vi "Word_OpenReference.vi"(5 "Template File Path":string="C:\\Teststand\\LVFiles\\Support\\Sertifika_Format.dotx", 7 "File Visible ?":bool=TRUE, 8 "error in (no error)":errorcluster) -> (0 "error out":errorcluster, 3 "report out":refnum<class "NI_report.lvclass">)   [LabVIEW 2014]
doc: "This VI demonstrates the use of ActiveX to write a table into a Microsoft Excel worksheet."
uses:
  <vilib>/Utility/NIReport.llb/NI_report.lvclass
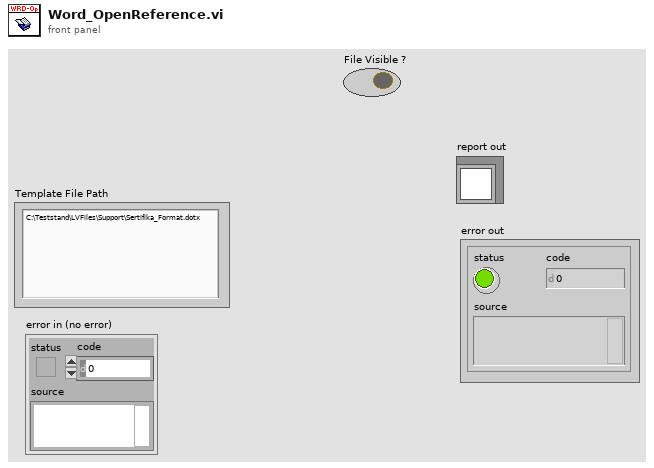
[diagram p1: front panel]
types:
  T1 = enum16{"Standard Report", "HTML", "Word", "Excel"}
  T2 = enum16{"maximized", "minimized", "normal", "no change"}
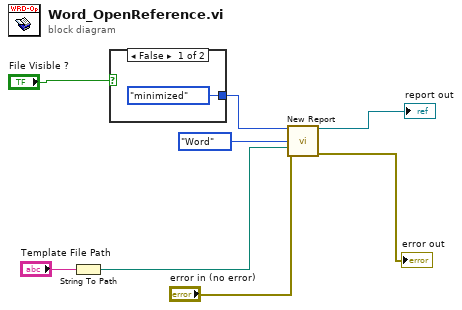
[diagram p0: block diagram]
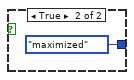
[diagram p2: hidden frame]
diagram:
  n1 = String To Path(string="Template File Path") -> (path=w4:path)
  n2 = case shown="False" "File Visible ?" {
    tunnel: [T2."minimized" ("window state (normal)") T2."maximized" ("window state (normal)")] -> w7
    frame False {
    }
    frame True {
    }
  }
  n3 = call <vilib>:"New Report.vi"("window state (normal)"=w7, "report type"=T1."Word", "template (empty)"=w4, "error in (no error)"="error in (no error)") -> ("report out"=→"report out":refnum<class "NI_report.lvclass">, "error out"=→"error out":errorcluster)  [unwired: 10 in]
